vi "Load Waveform Chart History - single plot.vi"(8 "error in (no error)":errorcluster, 10 "Plot GUI label":string, 11 "Father of all uServices in":refnum<class "Father of all uServices.lvclass">) -> (0 "error out":errorcluster, 2 "History Data - single plot":waveform(dbl)[](array[waveform]), 3 "Father of all uServices out":refnum<class "Father of all uServices.lvclass">)   [LabVIEW 2026, in "TALOS.lvlib" / "Father of all uServices.lvlib" / "Father of all uServices.lvclass"]
uses:
  Father of all uServices.lvclass
  Children Methods/Waveform Chart Class Reference Strict - single plot.ctl
  Ancestor/Ancestor/Ancestor.lvclass/Ancestor.ctl
  Support VIs/Generate Error.vi
  FGV/Error Memory/Get Error Description.vi
  Support VIs/Get PC name.vi
  Ancestor/Ancestor/Read ID.vi
  Support VIs/Get Class Name.vi
  FGV/Error Memory/Error Memory Core.vi
  <vilib>/AdvancedString/Delimited String to 1D String Array.vi
  <vilib>/AdvancedString/Delimited String to 1D String Array (string).vi
  Support VIs/Circus Root Path.vi
  FGV/Error Memory/Error Crt Lvl checker.vi
  FGV/Error Memory/Error Memory Core.vi/40c8088d-b597-4017-91af-faa98e00292e.vi
  FGV/Error Memory/Error Memory Core.vi/d4a3ab98-063c-4e44-b43d-fbdcfe6c2be2.vi
  <vilib>/Utility/file.llb/Read Delimited Spreadsheet (DBL).vi
  Support VIs/Global Memory.vi
  <vilib>/Utility/LVClass/Get LV Class Name.vi
  Support VIs/Is in Packed Library.vi
  Support VIs/TALOS Root path.vi
  Support VIs/Read CSV worksheet.vi
  Support VIs/Global Constants.vi
  <vilib>/Utility/error.llb/General Error Handler.vi
  Ancestor/Ancestor/Ancestor.lvclass
  <vilib>/Comparison/Equal/Equal Functor/Equal Functor.lvclass
  TALOS.lvlib
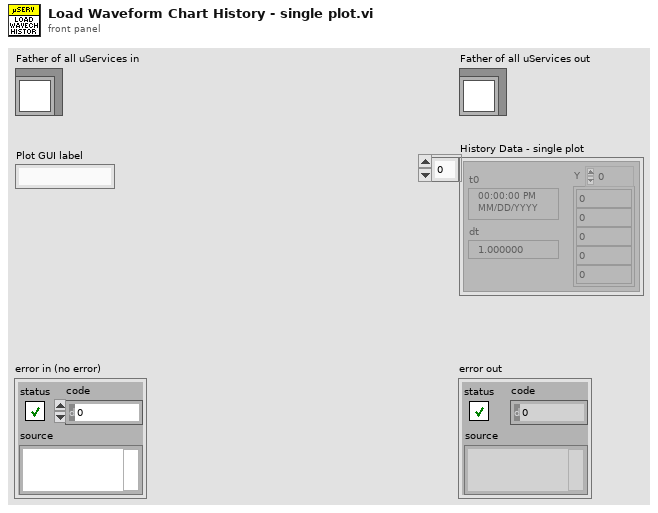
[diagram p1: front panel]
types:
  T1 = typedef "TALOS.lvlib/Father of all uServices.lvlib/Father of all uServices.lvclass/Waveform Chart Class Reference Strict - single plot.ctl" = refnum<vi>
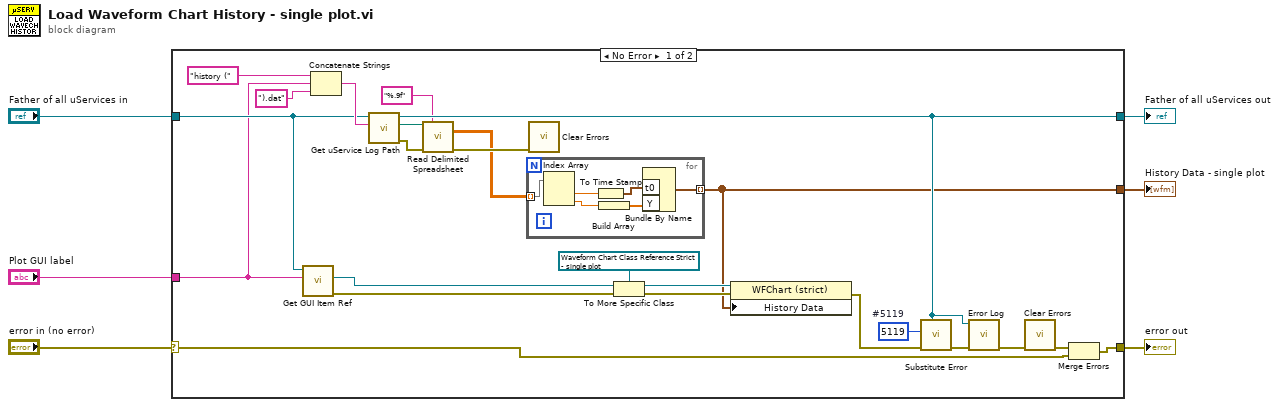
[diagram p0: block diagram]
diagram:
  n1 = case shown="No Error" "error in (no error)" {
    selector: "error in (no error)" -> [w8 w38]
    tunnel: [w9 w38] -> w5
    tunnel: [w24 w37] -> w3
    tunnel: "Father of all uServices in" -> [w16 w37]
    tunnel: "Plot GUI label" -> [w15 _]
    tunnel: [w10 _] -> w1
    frame No Error {
      w27 = 5119  # #5119
      n2 = call "Get GUI Item Ref.vi"("FP Item Name"=w15, "uService Template in"=w16) -> ("error out"=w13:errorcluster, "Ctl Refnum"=w14:refnum<vi>)  [unwired: 7 in, 1 out]
      n3 = Concatenate Strings("history (" ("string"), w15, ").dat" ("string")) -> (w28:string)
      n4 = call "Get uService Log Path.vi"("Log File Suffix"=w28, "Father of all uServices in"=w16) -> ("error out"=w18:errorcluster, "Log File Path"=w19:path, "Father of all uServices out"=w24:refnum<class "Father of all uServices.lvclass">)  [unwired: 7 in]
      n5 = call-poly <vilib>:"Read Delimited Spreadsheet.vi"("file path (dialog if empty)"=w19, "format (%.3f)"="%.9f", "error in (no error)"=w18) -> ("all rows"=w11:dbl[][], "error out"=w12:errorcluster)  [unwired: 7 in, 4 out]
      n6 = for {
        tunnel: w11 -> [w36] mode=indexing
        tunnel: [w34] -> w10 mode=indexing
        n7 = Index Array(array=w36) -> (element #1=w35:dbl, element #2=w31:dbl)  [unwired: 2 in]
        n8 = To Time Stamp(1:w35) -> (0:w33:timestamp)
        n9 = Build Array(w31) -> (w32:dbl[])
        n10 = Bundle By Name("t0"=w33, "Y"=w32) -> (w34:waveform(dbl))  [unwired: 1 in]
      }
      n11 = call <vilib>:"Clear Errors.vi"("error in (no error)"=w12) -> ()  [unwired: 5 in, 2 out]
      n12 = To More Specific Class(target class=T1 refnum ("WFChart Refnum"), reference=w14, error in=w13) -> (specific class reference=w21:T1, error out=w20:errorcluster)
      n13 = property class="WFChart (strict)"(reference=w21, error in=w20, "History Data"=w10) -> (error out=w26:errorcluster)  [unwired: 1 out]
      n14 = call "Substitute Error.vi"("LabVIEW Object"=w24, "error in (no error)"=w26, "Error Code"=w27) -> ("error out"=w25:errorcluster)  [unwired: 8 in]
      n15 = call "Error Log.vi"("error in (no error)"=w25, "Object in"=w24) -> ("error out"=w23:errorcluster)  [unwired: 9 in]
      n16 = call <vilib>:"Clear Errors.vi"("error in (no error)"=w23) -> ("error out"=w22:errorcluster)  [unwired: 5 in, 1 out]
      n17 = Merge Errors(w22, w8) -> (w9:errorcluster)
    }
    frame Error {
    }
  }
  "error out" <- w5
  "Father of all uServices out" <- w3
  "History Data - single plot" <- w1
